vi "DSF.Engine.BuilderManager.Set Builder FIFO.vi"(10 "Builder FIFO":refnum<k33>, 11 "Builder in":refnum<class "DSF.Engine.BuilderManager.lvclass">) -> (3 "Builder out":refnum<class "DSF.Engine.BuilderManager.lvclass">)   [LabVIEW 2017, in "DSF.Engine.lvlib" / "DSF.Engine.BuilderManager.lvclass"]
uses:
  DSF.Engine.BuilderManager.lvclass
  DSF.Engine.BuilderManager.lvclass/DSF.Engine.BuilderManager.ctl
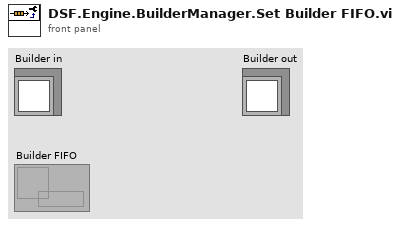
[diagram p1: front panel]
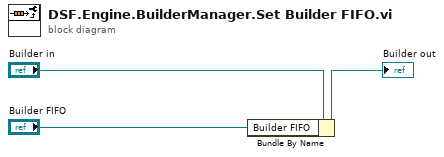
[diagram p0: block diagram]
diagram:
  n1 = Bundle By Name(cluster="Builder in", "Builder FIFO"="Builder FIFO") -> (→"Builder out":refnum<class "DSF.Engine.BuilderManager.lvclass">)
